vi "launch simple tcp listener.vi"(4 "data":variant[](array[variant]), 6 "terminals":string[](array[string]), 8 "error in":errorcluster, 10 "callback VI Refnum":refnum<vi>, 11 "port":u16) -> (0 "error out":errorcluster, 3 "shutdown notifier":refnum<notifier>)   [LabVIEW 2013]
doc: "This VI launches a TCP server which accepts incoming connections and launches a reentrant handler VI specified by the callback refnum. This VI requires that the callback has a front panel control titled \"connection\" of type tcp refnum."
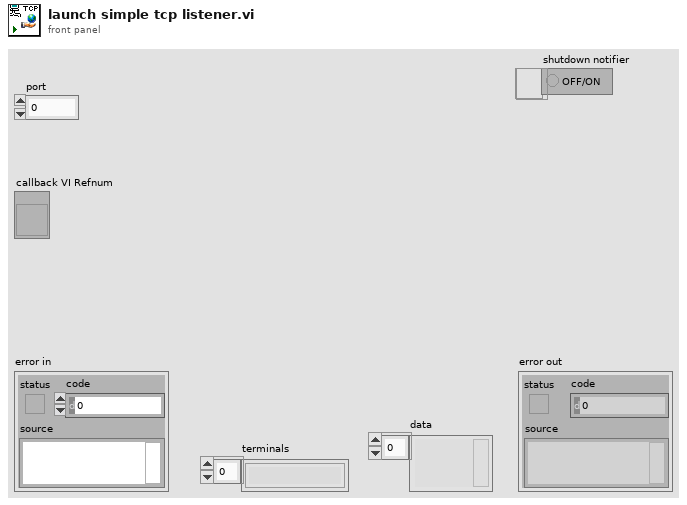
[diagram p1: front panel]
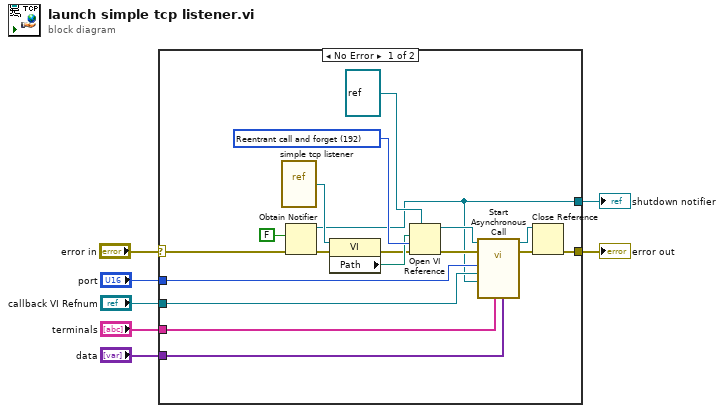
[diagram p0: block diagram]
diagram:
  n1 = case shown="No Error" "error in" {
    selector: "error in" -> [w11 w26]
    tunnel: [w16 w26] -> w6
    tunnel: "port" -> [w14 _]
    tunnel: "callback VI Refnum" -> [w15 _]
    tunnel: "terminals" -> [w12 _]
    tunnel: "data" -> [w13 _]
    tunnel: [w8 _] -> w1
    frame No Error {
      w25 = 192 items=["Prepare to call and forget"=128, "Prepare to call and collect"=256, "Reentrant call and forget"=192, "Reentrant call and collect"=320] ("VI Server Options")
      n2 = vi-ref "simple tcp listener.vi"() -> (w22:refnum<vi>)
      n3 = Obtain Notifier(notification data type=FALSE, error in (no error)=w11) -> (notifier out=w8:refnum<notifier>, error out=w10:errorcluster)  [unwired: 2 in, 1 out]
      n4 = property class="VI"(reference=w22, error in=w10) -> (error out=w23:errorcluster, "Path"=w24:path)  [unwired: 1 out]
      n5 = Open VI Reference(type specifier VI Refnum (for type only)=refnum<vi> refnum, vi path=w24, options=w25, error in (no error)=w23) -> (vi reference=w20:refnum<vi>, error out=w21:errorcluster)  [unwired: 2 in]
      n6 = call-by-ref "Start Asynchronous Call"(reference=w20, error in=w21, "data"=w13, "terminals"=w12, "stop notification"=w8, "callback VI Refnum"=w15, "port"=w14) -> (reference out=w17:refnum<vi>, error out=w18:errorcluster)  [unwired: 7 in]
      n7 = Close Reference(reference=w17, error in (no error)=w18) -> (error out=w16:errorcluster)
    }
    frame Error {
    }
  }
  "error out" <- w6
  "shutdown notifier" <- w1
